vi "close_connection.vi"(0 "reference (in)":refnum<class "_Controller.lvclass">, 5 "error in (no error)":errorcluster) -> (14 "reference (out)":refnum<class "_Controller.lvclass">, 19 "error out":errorcluster)   [LabVIEW 2020, in "classes.lvlib" / "_Controller.lvclass"]
doc: "Closes the USB connect to the referenced device.\n\nImplementss the USB Communication API function \"fnPerformaxComClose()'.\n\nProduced By:\n\n<B>Kod Integrations, LLC</B>\n4835 Marianne Drive\nMount Airy, MD 21771\nhttp://www.kodintegrations.com\nemail: info@kodintegrations.com\nphone: (240) 687-1288"
uses:
  _Controller.lvclass
  models.ctl
  _Controller.lvclass/_Controller.ctl
  error_actions.ctl
  common.lvlib
  PerformaxCom.dll
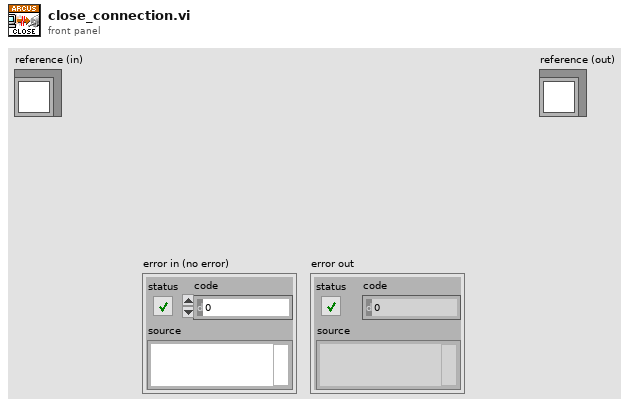
[diagram p1: front panel]
types:
  T1 = typedef "common.lvlib/models.ctl" = enum16{"<unrecognized>", "ACE-SDC", "ACE-SDE", "ACE-SXC", "ACE-SXE", "DMX-CAN", "DMX-J-SA", "DMX-K-SA", "DMX-UMD", "PMX-2ED-SA", "PMX-2EX-SA", "PMX-4CX-SA", "PMX-4EX-SA"}
  T2 = typedef "common.lvlib/error_actions.ctl" = enum16{"clearBuff", "closeRef", "nodeErr", "noDeviceInfo", "noDevices", "openRef", "sendReceive", "setTimeouts", "unknown"}
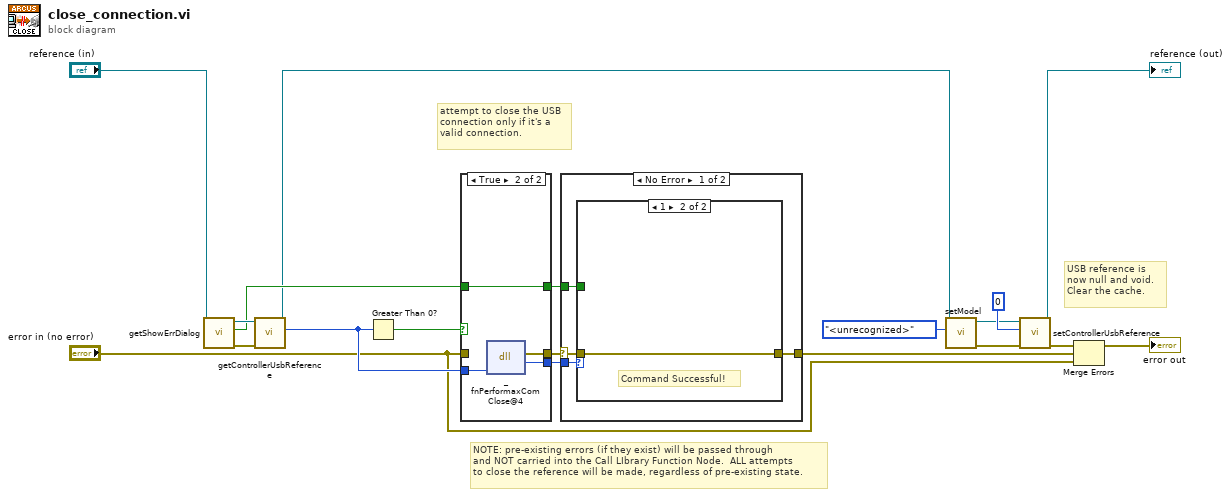
[diagram p0: block diagram]
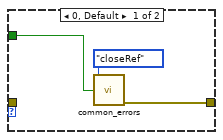
[diagram p2: hidden frame]
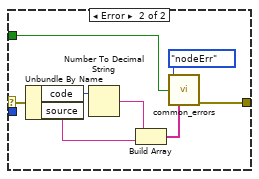
[diagram p3: hidden frame]
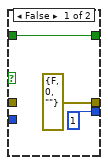
[diagram p4: hidden frame]
diagram:
  # "attempt to close the USB\nconnection only if it's a\nvalid connection."
  # "NOTE: pre-existing errors (if they exist) will be passed through\nand NOT carried into the Call LIbrary Function Node.  ALL attempts\nto close the reference will be made, regardless of pre-existing state."
  # "USB reference is \nnow null and void.\nClear the cache."
  n1 = call "getShowErrDialog.vi"("reference (in)"="reference (in)") -> ("error out"=w15:errorcluster, "showErrDialog"=w6:bool, "reference (out)"=w18:refnum<class "_Controller.lvclass">)  [unwired: 8 in]
  n2 = call "getControllerUsbReference.vi"("error in (no error)"=w15, "reference (in)"=w18) -> ("reference"=w7:i32, "reference (out)"=w3:refnum<class "_Controller.lvclass">)  [unwired: 7 in, 1 out]
  n3 = Greater Than 0?(x=w7) -> (x > 0?=w12:bool)
  n4 = case shown="True" w12 {
    tunnel: [1 w26] -> w10
    tunnel: [errorcluster {"status"=FALSE, "code"=0, "source"=""} ("error out") w24] -> w9
    tunnel: "error in (no error)" -> [_ _]
    tunnel: w7 -> [_ w25]
    tunnel: [w21 w23] -> w11
    tunnel: w6 -> [w21 w23]
    frame False {
    }
    frame True {
      n5 = dll-call lib="PerformaxCom.dll" fn="_fnPerformaxComClose@4"("reference"=w25) -> (error out=w24:errorcluster, "return type"=w26:i32)  [unwired: 4 in, 1 out]
    }
  }
  n6 = case shown="No Error" w9 {
    selector: w9 -> [w27 w39]
    tunnel: [w30 w42] -> w8
    tunnel: w10 -> [w29 _]
    tunnel: w11 -> [w28 w41]
    frame No Error {
      n7 = case shown="1" w29 {
        tunnel: [w32 w34] -> w30
        tunnel: w27 -> [_ w34]
        tunnel: w28 -> [w31 _]
        frame 0, Default {
          n8 = call "common_errors.vi"("common_errors"=error_actions."closeRef" ("errors"), "dialog? (T)"=w31) -> ("error out"=w32:errorcluster)  [unwired: 13 in]
        }
        frame 1 {
          # "Command Successful!"
        }
      }
    }
    frame Error {
      n9 = Unbundle By Name(w39) -> ("code"=w38:i32, "source"=w36:string)
      n10 = Number To Decimal String(number=w38) -> (decimal integer string=w37:string)  [unwired: 1 in]
      n11 = Build Array(w37, w36) -> (w35:string[])
      n12 = call "common_errors.vi"("common_errors"=error_actions."nodeErr" ("errors"), "dialog? (T)"=w41, "supp_text"=w35) -> ("error out"=w42:errorcluster)  [unwired: 12 in]
    }
  }
  n13 = call "setModel.vi"("model"=models."<unrecognized>", "reference (in)"=w3) -> ("error out"=w4:errorcluster, "reference (out)"=w2:refnum<class "_Controller.lvclass">)  [unwired: 8 in]
  n14 = call "setControllerUsbReference.vi"("error in (no error)"=w4, "reference"=0, "reference (in)"=w2) -> ("error out"=w14:errorcluster, "reference (out)"=→"reference (out)":refnum<class "_Controller.lvclass">)  [unwired: 7 in]
  n15 = Merge Errors(w14, w8, "error in (no error)") -> (→"error out":errorcluster)
